vi "Build Context.vi"(9 "Context Value":string, 10 "Context Name":T2 items=["Method Name", "Parameter Name", "VI Name", "Control Name", "Proxy Dll Path", "Project Library Name"]) -> (1 "Context":T1 {"name" items=["Method Name", "Parameter Name", "VI Name", "Control Name", "Proxy Dll Path", "Project Library Name"]})   [LabVIEW 2017, in "WebServiceImporter.lvlib" / "Error Handling.lvlib"]
uses:
  <vilib>/Platform/WebService/Error Handling/Error Handling.lvlib
  <vilib>/Platform/WebService/Error Handling/Error/Context Name.ctl
  <vilib>/Platform/WebService/Error Handling/Error/Context.ctl
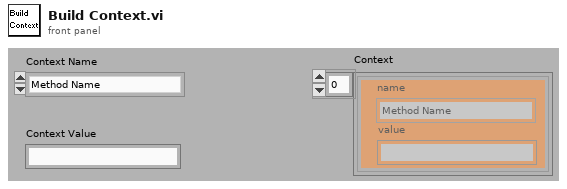
[diagram p1: front panel]
types:
  T1 = typedef "WebServiceImporter.lvlib/Error Handling.lvlib/Context.ctl" = cluster{"name":T2, "value":string}[]
  T2 = typedef "WebServiceImporter.lvlib/Error Handling.lvlib/Context Name.ctl" = u16
  T3 = cluster{"Context Name":T2, "Context Value":string}
  T4 = cluster{"Context Name":T2, "Context Value":string}[]
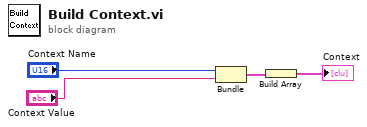
[diagram p0: block diagram]
diagram:
  n1 = Bundle("Context Name"="Context Name", "Context Value"="Context Value") -> (w2:T3)  [unwired: 1 in]
  n2 = Build Array(w2) -> (→"Context":T4)
